vi "VI Tree.vi"   [LabVIEW 2011, in "Template - Power Meter.lvlib"]
doc: "This is the instrument driver for the <INSTRUMENT NAME>. The VI Tree displays all the user-callable VIs of the instrument driver in an organized table."
uses:
  <instrlib>/_Template - Power Meter/Template - Power Meter.lvlib
panel:
  # "(c) 2009 <Enter Company Name Here>.  ALL RIGHTS RESERVED."
  # "SEE DIAGRAM\nFOR VI TREE."
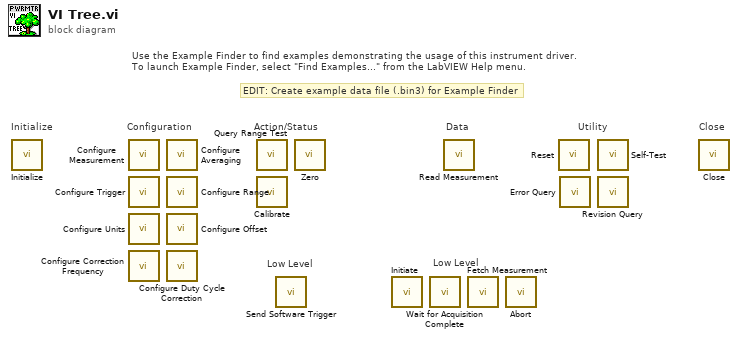
[diagram p0: block diagram]
diagram:
  # "Low Level"
  # "Low Level"
  # "EDIT: Create example data file (.bin3) for Example Finder"
  # "Use the Example Finder to find examples demonstrating the usage of this instrument driver.\nTo launch Example Finder, select \"Find Examples...\" from the LabVIEW Help menu."
  # "Configuration"
  # "Utility"
  # "Data"
  # "Action/Status"
  # "Close"
  # "Initialize"
  n1 = call <instrlib>:"Initialize.vi"() -> ()  [unwired: 10 in, 2 out]
  n2 = call <instrlib>:"Configure Measurement.vi"() -> ()  [unwired: 14 in, 2 out]
  n3 = call <instrlib>:"Configure Trigger.vi"() -> ()  [unwired: 14 in, 2 out]
  n4 = call <instrlib>:"Configure Units.vi"() -> ()  [unwired: 10 in, 2 out]
  n5 = call <instrlib>:"Configure Correction Frequency.vi"() -> ()  [unwired: 10 in, 2 out]
  n6 = call <instrlib>:"Configure Averaging.vi"() -> ()  [unwired: 14 in, 2 out]
  n7 = call <instrlib>:"Configure Range.vi"() -> ()  [unwired: 10 in, 2 out]
  n8 = call <instrlib>:"Configure Offset.vi"() -> ()  [unwired: 10 in, 2 out]
  n9 = call <instrlib>:"Configure Duty Cycle Correction.vi"() -> ()  [unwired: 10 in, 2 out]
  n10 = call <instrlib>:"Query Range Test.vi"() -> ()  [unwired: 9 in, 3 out]
  n11 = call <instrlib>:"Calibrate.vi"() -> ()  [unwired: 10 in, 2 out]
  n12 = call <instrlib>:"Send Software Trigger.vi"() -> ()  [unwired: 10 in, 2 out]
  n13 = call <instrlib>:"Zero.vi"() -> ()  [unwired: 10 in, 2 out]
  n14 = call <instrlib>:"Initiate.vi"() -> ()  [unwired: 10 in, 2 out]
  n15 = call <instrlib>:"Wait for Acquisition Complete.vi"() -> ()  [unwired: 10 in, 2 out]
  n16 = call <instrlib>:"Read Measurement.vi"() -> ()  [unwired: 9 in, 3 out]
  n17 = call <instrlib>:"Fetch Measurement.vi"() -> ()  [unwired: 9 in, 3 out]
  n18 = call <instrlib>:"Abort.vi"() -> ()  [unwired: 10 in, 2 out]
  n19 = call <instrlib>:"Reset.vi"() -> ()  [unwired: 10 in, 2 out]
  n20 = call <instrlib>:"Error Query.vi"() -> ()  [unwired: 8 in, 4 out]
  n21 = call <instrlib>:"Self-Test.vi"() -> ()  [unwired: 8 in, 4 out]
  n22 = call <instrlib>:"Revision Query.vi"() -> ()  [unwired: 8 in, 4 out]
  n23 = call <instrlib>:"Close.vi"() -> ()  [unwired: 11 in, 1 out]
